vi "LabVIEW Environments Installed (Win10).vi"() -> (1 "Current LabVIEW x64 Index":i32, 2 "Current LabVIEW x86 Index":i32, 3 "LabVIEW Applications Installed":T1(array[cluster]))   [LabVIEW 2020]
doc: "Created by Ryan Pacini"
uses:
  <vilib>/registry/registry.llb/Registry RtKey.ctl
  <vilib>/registry/registry.llb/Registry SAM.ctl
  <vilib>/registry/registry.llb/Registry View.ctl
  <vilib>/registry/registry.llb/Read Registry Value Simple STR.vi
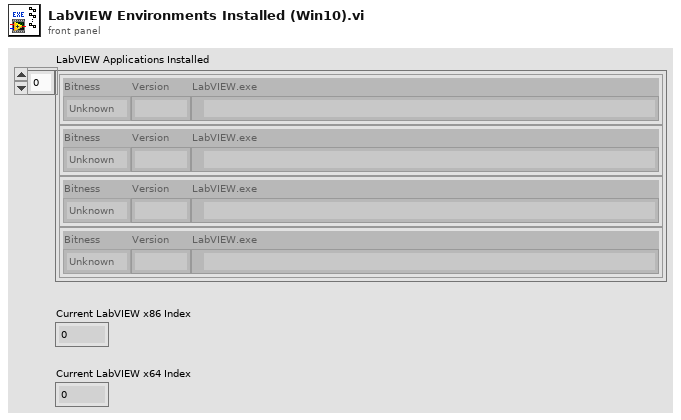
[diagram p1: front panel]
types:
  T1 = cluster{"Bitness":enum8{"Unknown", "x86", "x64"}, "Version":string, "LabVIEW.exe":path}[]
  T2 = typedef "Registry View.ctl" = u16
  T3 = typedef "Registry SAM.ctl" = enum32{"KEY_QUERY_VALUE", "KEY_SET_VALUE", "KEY_CREATE_SUB_KEY", "KEY_ENUMERATE_SUB_KEYS", "KEY_NOTIFY", "KEY_CREATE_LINK", "KEY_READ", "KEY_WRITE", "KEY_ALL_ACCESS", "KEY_READ | KEY_WRITE"}
  T4 = typedef "Registry RtKey.ctl" = enum32{"HKEY_CLASSES_ROOT", "HKEY_CURRENT_USER", "HKEY_LOCAL_MACHINE", "HKEY_USERS", "HKEY_PERFORMANCE_DATA", "HKEY_CURRENT_CONFIG", "HKEY_DYN_DATA"}
  T5 = cluster{"Bitness":enum8{"Unknown", "x86", "x64"}, "Version":string, "LabVIEW.exe":path}
  T6 = enum16{"open", "replace", "create", "open or create", "replace or create", "replace or create with confirmation"}
  T7 = typedef "Registry refnum.ctl" = refnum<k1>
  T8 = cluster{"numSubKeys":i32, "maxSubKeyLen":i32, "maxSubKeyClassLen":i32}
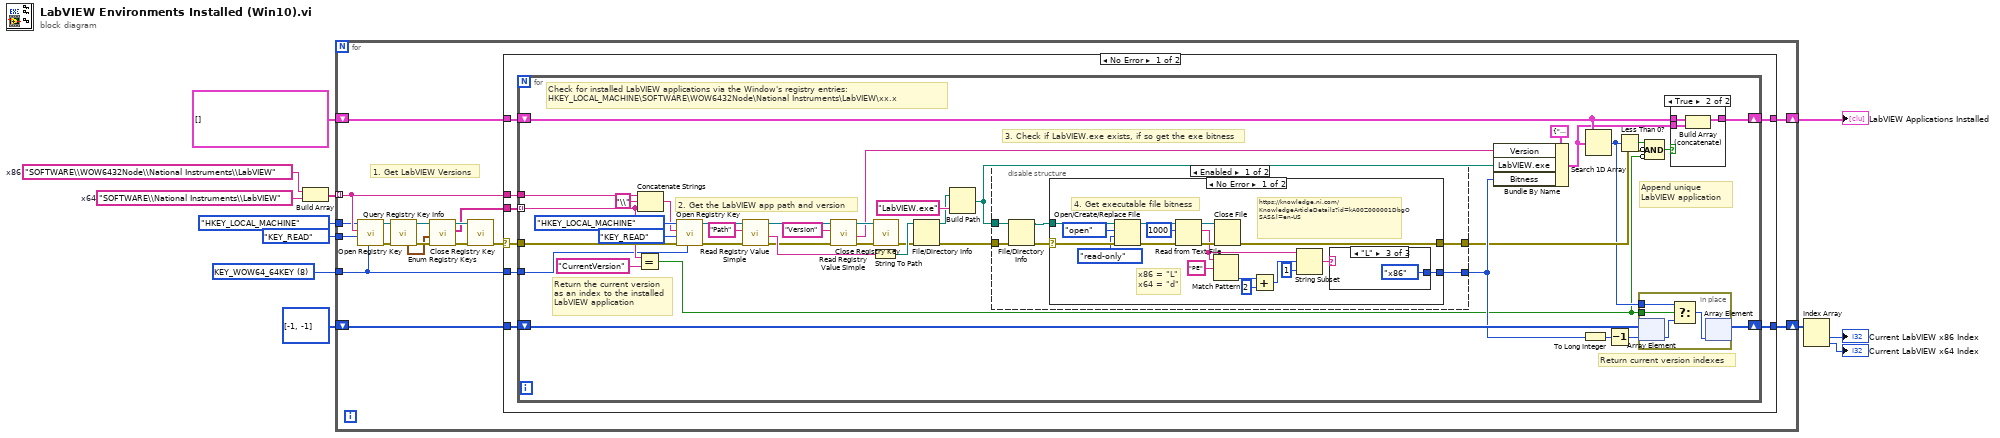
[diagram p0: block diagram]
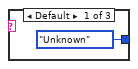
[diagram p2: hidden frame]
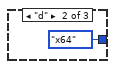
[diagram p3: hidden frame]
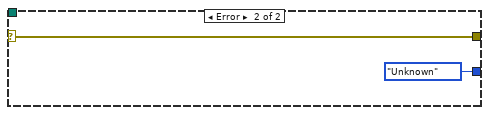
[diagram p4: hidden frame]
diagram:
  w1 = T2 8 items=["Default"=0, "KEY_WOW64_64KEY"=8, "KEY_WOW64_32KEY"=9] ("registry view")
  w5 = "SOFTWARE\\National Instruments\\LabVIEW"  # x64
  w12 = "SOFTWARE\\WOW6432Node\\National Instruments\\LabVIEW"  # x86
  n1 = Build Array(w12, w5) -> (w6:string[])
  n2 = for {
    tunnel: w6 -> [w21] mode=indexing
    shift-right: [w17] -> w9
    shift-left: T1 [] ("LabVIEW Applications Installed") -> [w18]
    shift-right: [w19] -> w11
    shift-left: i32[] [-1, -1] ("index of element") -> [w16]
    tunnel: Registry_RtKey."HKEY_LOCAL_MACHINE" ("root key (HKEY_LOCAL_MACHINE)") -> [w15]
    tunnel: Registry_SAM."KEY_READ" ("security access mask (KEY_READ | KEY_WRITE)") -> [w14]
    tunnel: w1 -> [w13]
    # "1. Get LabVIEW Versions"
    n3 = call <vilib>:"Open Registry Key.vi"("registry view"=w13, "security access mask (KEY_READ | KEY_WRITE)"=w14, "subkey"=w21, "root key (HKEY_LOCAL_MACHINE)"=w15) -> ("error out"=w27:errorcluster, "refnum out"=w28:T7)  [unwired: 6 in]
    n4 = call <vilib>:"Query Registry Key Info.vi"("error in (no error)"=w27, "refnum"=w28) -> ("error out"=w25:errorcluster, "refnum out"=w26:T7, "subkey info"=w24:T8)  [unwired: 5 in, 2 out]
    n5 = call <vilib>:"Enum Registry Keys.vi"("error in (no error)"=w25, "subkey info"=w24, "refnum"=w26) -> ("error out"=w29:errorcluster, "subkeys"=w20:string[], "refnum out"=w22:T7)  [unwired: 6 in]
    n6 = call <vilib>:"Close Registry Key.vi"("error in (no error)"=w29, "refnum"=w22) -> ("error out"=w23:errorcluster)  [unwired: 5 in]
    n7 = case shown="No Error" w23 {
      selector: w23 -> [w37 _]
      tunnel: w21 -> [w36 _]
      tunnel: w20 -> [w35 _]
      tunnel: [w34 w116] -> w17
      tunnel: [w33 w115] -> w19
      tunnel: w18 -> [w32 w116]
      tunnel: w16 -> [w31 w115]
      tunnel: w13 -> [w30 _]
      frame No Error {
        n8 = for {
          tunnel: w36 -> [w70]
          tunnel: w35 -> [w41] mode=indexing
          tunnel: w37 -> [w75]
          shift-right: [w66] -> w34
          shift-left: w32 -> [w67]
          shift-right: [w54] -> w33
          shift-left: w31 -> [w55]
          tunnel: w30 -> [w38]
          # "Return the current version\nas an index to the installed\nLabVIEW application"
          # "Append unique\nLabVIEW application"
          # "Check for installed LabVIEW applications via the Window's registry entries:\nHKEY_LOCAL_MACHINE\\SOFTWARE\\WOW6432Node\\National Instruments\\LabVIEW\\xx.x"
          # "Return current version indexes"
          # "3. Check if LabVIEW.exe exists, if so get the exe bitness"
          # "2. Get the LabVIEW app path and version"
          n9 = Equal?(x=w41, y="CurrentVersion" ("x")) -> (x = y?=w40:bool)
          n10 = Concatenate Strings(w70, "\\" ("string"), w41) -> (w47:string)
          n11 = call <vilib>:"Open Registry Key.vi"("registry view"=w38, "error in (no error)"=w75, "security access mask (KEY_READ | KEY_WRITE)"=Registry_SAM."KEY_READ", "subkey"=w47, "root key (HKEY_LOCAL_MACHINE)"=Registry_RtKey."HKEY_LOCAL_MACHINE") -> ("error out"=w74:errorcluster, "refnum out"=w73:T7)  [unwired: 5 in]
          n12 = call-poly <vilib>:"Read Registry Value Simple.vi"("error in (no error)"=w74, "value"="Path", "refnum"=w73) -> ("error out"=w51:errorcluster, "String/Binary data"=w57:string, "refnum out"=w45:T7)  [unwired: 3 in, 1 out]
          n13 = call-poly <vilib>:"Read Registry Value Simple.vi"("error in (no error)"=w51, "value"="Version", "refnum"=w45) -> ("error out"=w46:errorcluster, "String/Binary data"=w42:string, "refnum out"=w44:T7)  [unwired: 3 in, 1 out]
          n14 = String To Path(string=w57) -> (path=w72:path)
          n15 = call <vilib>:"Close Registry Key.vi"("error in (no error)"=w46, "refnum"=w44) -> ("error out"=w68:errorcluster)  [unwired: 5 in]
          n16 = File/Directory Info(path=w72, error in=w68) -> (path out=w64:path, error out=w63:errorcluster)  [unwired: 5 out]
          n17 = Build Path(base path=w64, name or relative path="LabVIEW.exe") -> (appended path=w39:path)
          n18 = disable-structure shown="Enabled" {
            disable-tunnel: w63 -> [w82 w106]
            disable-tunnel: [w80 _] -> w53
            disable-tunnel: [w79 w106] -> w50
            disable-tunnel: w39 -> [w78 _]
            frame Enabled {
              n19 = File/Directory Info(path=w78, error in=w82) -> (path out=w77:path, error out=w81:errorcluster)  [unwired: 5 out]
              n20 = case shown="No Error" w81 {
                selector: w81 -> [w100 w105]
                tunnel: [w83 enum8{"Unknown", "x86", "x64"}."Unknown" ("Bitness")] -> w80
                tunnel: [w99 w105] -> w79
                tunnel: w77 -> [w98 _]
                frame No Error {
                  # "x86 = \"L\"\nx64 = \"d\""
                  # "4. Get executable file bitness"
                  # "https://knowledge.ni.com/KnowledgeArticleDetails?id=kA00Z000001DbgOSAS&l=en-US"
                  n21 = Open/Create/Replace File(file path (use dialog)=w98, error in=w100, operation (0:open)=T6."open", access (0:read/write)=enum16{"read/write", "read-only", "write-only"}."read-only") -> (refnum out=w97:refnum<file>, error out=w96:errorcluster)  [unwired: 2 in, 1 out]
                  n22 = Read from Text File(file (use dialog)=w97, count=1000, error in=w96) -> (refnum out=w94:refnum<file>, text=w89:string, error out=w95:errorcluster)  [unwired: 1 in, 1 out]
                  n23 = Match Pattern(string=w89, regular expression="PE") -> (offset past match=w91:i32)  [unwired: 1 in, 3 out]
                  n24 = Close File(refnum=w94, error in=w95) -> (error out=w99:errorcluster)  [unwired: 1 out]
                  n25 = Add(x=w91, y=2) -> (x+y=w88:i32)
                  n26 = String Subset(string=w89, offset (0)=w88, length (rest)=1 ("length (rest)")) -> (substring=w84:string)
                  n27 = case shown="\"L\"" w84 {
                    tunnel: [enum8{"Unknown", "x86", "x64"}."Unknown" ("Bitness") enum8{"Unknown", "x86", "x64"}."x64" ("Bitness") enum8{"Unknown", "x86", "x64"}."x86" ("Bitness")] -> w83
                    frame Default {
                    }
                    frame "d" {
                    }
                    frame "L" {
                    }
                  }
                }
                frame Error {
                }
              }
            }
            frame Disabled {
            }
          }
          n28 = Bundle By Name(cluster=T5 {"Bitness"=enum."Unknown", "Version"="", "LabVIEW.exe"=path ""} ("LabVIEW Application"), "Version"=w42, "LabVIEW.exe"=w39, "Bitness"=w53) -> (w60:T5)
          n29 = To Long Integer(number=w53) -> (32bit integer=w52:i32)
          n30 = Search 1D Array(1D array=w67, element=w60) -> (index of element=w49:i32)  [unwired: 1 in]
          n31 = Decrement(x=w52) -> (x-1=w48:i32)
          n32 = Less Than 0?(x=w49) -> (x < 0?=w62:bool)
          n33 = in-place {
            in-place-border: w49 -> [w110]
            in-place-border: w40 -> [w109]
            n34 = in-place-array #1(w55, w48) -> (w108:i32)
            n35 = Select(t=w110, s=w109, f=w108) -> (s? t:f=w107:i32)
            n36 = in-place-array #1(w107) -> (w54:i32[])  [unwired: 1 out]
          }
          n37 = Compound Arithmetic op=AND(w62, invert w50, invert w40) -> (w61:bool)
          n38 = case shown="True" w61 {
            tunnel: w67 -> [w111 w114]
            tunnel: w60 -> [_ w113]
            tunnel: [w111 w112] -> w66
            frame False {
            }
            frame True {
              n39 = Build Array (concatenate)(w114, w113) -> (w112:T1)
            }
          }
        }
      }
      frame Error {
      }
    }
  }
  "LabVIEW Applications Installed" <- w9
  n40 = Index Array(array=w11) -> (element #1=→"Current LabVIEW x86 Index":i32, element #2=→"Current LabVIEW x64 Index":i32)  [unwired: 2 in]
